vi "Save Notebook Themes.vi"(8 "Error In":errorcluster) -> (0 "error out":errorcluster, 1 "cancelled":bool, 3 "Save File Path":path, 4 "Message":string)   [LabVIEW 2021, in "Notebook.lvlib"]
uses:
  Notebook.lvlib
  Notebook Parameters List.ctl
  Notebook Theme.ctl
  Rich Text Box/Named Text Style.ctl
  Rich Text Box/Text Formatting.ctl
  Rich Text Box/Text Colors.ctl
  Rich Text Box/Text Style.ctl
  Rich Text Box/Text Alignment.ctl
  ad7bbb2b-3b95-4723-af1b-4fb2c45ed1f4.vi
  <vilib>/JDP Science/JSONtext/Variant to JSON Text.vi
  <vilib>/JDP Science/JSONtext/LVClass Serializer/JSONtext LVClass Serializer.lvclass
  Rich Text Box/Rich Text Box.lvlib
  Files/Files.lvlib
panel:
  # "see the License on the block diagram (Ctrl+E or Window:Show Block Diagram)"
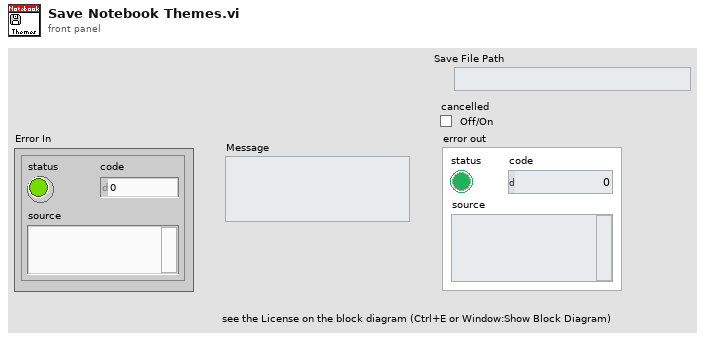
[diagram p1: front panel]
types:
  T1 = typedef "Notebook.lvlib/Notebook Theme.ctl" = cluster{"Theme Name":string, "[Named Text Styles]":T2[], "Page Color":T4}
  T2 = typedef "Notebook.lvlib/Named Text Style.ctl" = cluster{"Text Formatting":T3, "Text Style Name":string}
  T3 = typedef "Rich Text Box.lvlib/Text Formatting.ctl" = cluster{"Font":string, "Text Color":T4, "Background Color":T4, "Style":T5, "Font Size":dbl, "Alignment":T6}
  T4 = typedef "Rich Text Box.lvlib/Text Colors.ctl" = enum16{"Unchanged", "Black", "Blue", "Cyan", "Maroon", "Gray", "Violet", "Green", "Light Green", "Orange", "Yellow", "Magenta", "Red", "White"}
  T5 = typedef "Rich Text Box.lvlib/Text Style.ctl" = enum16{"Regular", "Bold", "Italic", "Underline", "Strikeout"}
  T6 = typedef "Rich Text Box.lvlib/Text Alignment.ctl" = enum16{"Left", "Right", "Center"}
  T7 = typedef "Notebook.lvlib/Notebook Parameters List.ctl" = enum16{"First Opening?", "Saved Notebook?", "Saved Notebook Path", "Beep on Error?", "Notebook Themes", "Current Theme Name"}
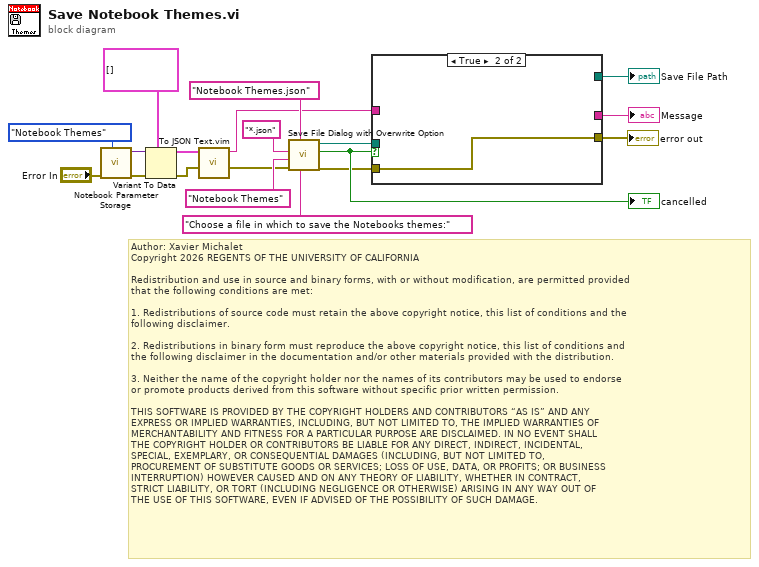
[diagram p0: block diagram]
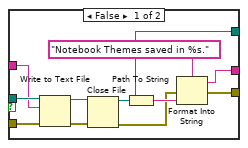
[diagram p2: hidden frame]
diagram:
  # "Author: Xavier Michalet\nCopyright 2026 REGENTS OF THE UNIVERSITY OF CALIFORNIA\n\nRedistribution and use in source and binary forms, with or without modification, are permitted provided\nthat the following conditions are met:\n\n1. Redistributions of source code must retain the above copyright notice, this list of conditions and the\nfollowing disclaimer.\n\n2. Redistributions in binary form must reproduce the above copyright notice, this list of conditions and\nthe following disclaimer in the documentation and/or other materials provided with the distribution.\n\n3. Neither the name of the copyright holder nor the names of its contributors may be used to endorse \nor promote products derived from this software without specific prior written permission.\n\nTHIS SOFTWARE IS PROVIDED BY THE COPYRIGHT HOLDERS AND CONTRIBUTORS “AS IS” AND ANY \nEXPRESS OR IMPLIED WARRANTIES, INCLUDING, BUT NOT LIMITED TO, THE IMPLIED WARRANTIES OF\nMERCHANTABILITY AND FITNESS FOR A PARTICULAR PURPOSE ARE DISCLAIMED. IN NO EVENT SHALL\nTHE COPYRIGHT HOLDER OR CONTRIBUTORS BE LIABLE FOR ANY DIRECT, INDIRECT, INCIDENTAL, \nSPECIAL, EXEMPLARY, OR CONSEQUENTIAL DAMAGES (INCLUDING, BUT NOT LIMITED TO, \nPROCUREMENT OF SUBSTITUTE GOODS OR SERVICES; LOSS OF USE, DATA, OR PROFITS; OR BUSINESS\nINTERRUPTION) HOWEVER CAUSED AND ON ANY THEORY OF LIABILITY, WHETHER IN CONTRACT, \nSTRICT LIABILITY, OR TORT (INCLUDING NEGLIGENCE OR OTHERWISE) ARISING IN ANY WAY OUT OF\nTHE USE OF THIS SOFTWARE, EVEN IF ADVISED OF THE POSSIBILITY OF SUCH DAMAGE."
  n1 = call "Notebook Parameter Storage.vi"("Notebook Parameter List"=Notebook_Parameters_List."Notebook Themes", "Error In"="Error In") -> ("Error Out"=w8:errorcluster, "Data out"=w7:variant)  [unwired: 8 in]
  n2 = Variant To Data(error in=w8, type=T1[] [] ("Array"), Variant=w7) -> (data=w10:T1[], error out=w11:errorcluster)
  n3 = call "To JSON Text.vim"("error in (no error)"=w11, "Anything"=w10) -> ("error out"=w12:errorcluster, "<JSON>"=w3:string)  [unwired: 8 in]
  n4 = call "Save File Dialog with Overwrite Option.vi"("prompt"="Choose a file in which to save the Notebooks themes:" ("prompt (Choose or enter file path)"), "Default Name"="Notebook Themes.json", "error in (no error)"=w12, "pattern label"="Notebook Themes", "pattern (all files)"="*.json") -> ("error out"=w13:errorcluster, "cancelled"=w19:bool, "selected path"=w14:path)  [unwired: 3 in, 1 out]
  "cancelled" <- w19
  n5 = case shown="True" w19 {
    tunnel: w13 -> [w25 w31]
    tunnel: w14 -> [w24 _]
    tunnel: [w23 w31] -> w5
    tunnel: w3 -> [w22 _]
    tunnel: [w21 _] -> w2
    tunnel: [w20 _] -> w1
    frame False {
      n6 = Write to Text File(file (use dialog)=w24, text=w22, error in=w25) -> (refnum out=w30:refnum<file>, error out=w29:errorcluster)  [unwired: 1 in, 1 out]
      n7 = Close File(refnum=w30, error in=w29) -> (path=w20:path, error out=w26:errorcluster)
      n8 = Path To String(path=w20) -> (string=w28:string)
      n9 = Format Into String(format string="Notebook Themes saved in %s.", error in=w26, w28) -> (resulting string=w21:string, error out=w23:errorcluster)  [unwired: 1 in]
    }
    frame True {
    }
  }
  "error out" <- w5
  "Message" <- w2
  "Save File Path" <- w1
